vi "Localization - Read and Parse File.vi"(8 "Error In":errorcluster, 9 "Full File Contents in":string[][](array[string]), 10 "Localization File Path":path=path "C:/Apps/Dev/CMC Internal/Team Tools/Development/Composite Controls/Test VI/INI Files/Test.ini" caption="Localization File for Referenced VI", 11 "VI Reference":refnum<vi>) -> (0 "Error Out":errorcluster, 1 "Full File Contents out":string[][](array[string]), 2 "Controls Not Present":string[](array[string]), 3 "Array":refnum<class "Control Info.lvclass">[](array[class]))   [LabVIEW 2017, in "Localization.lvlib"]
uses:
  Localization.lvlib
  Control Info/Control Info.lvclass
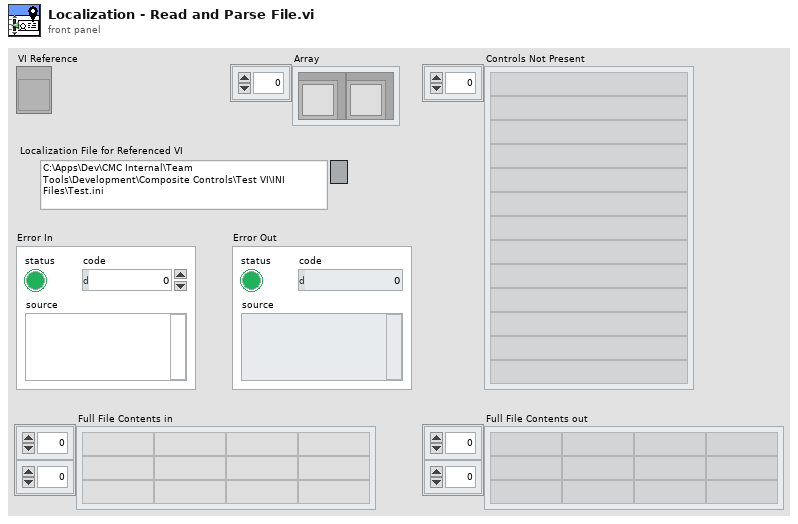
[diagram p1: front panel]
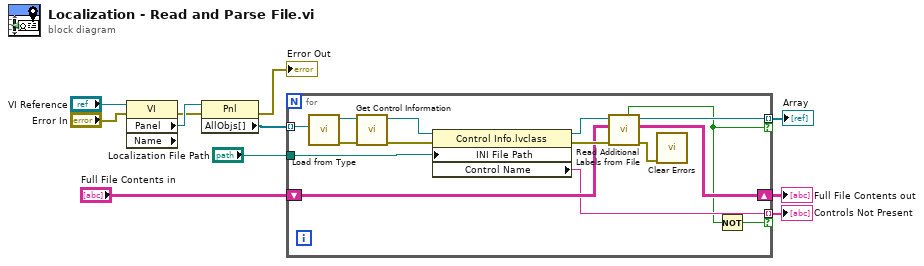
[diagram p0: block diagram]
diagram:
  n1 = property class="VI" props=["Panel", "Name"](reference="VI Reference", error in="Error In") -> (error out=w7:errorcluster, "Panel"=w8:refnum<vi>)  [unwired: 2 out]
  n2 = property class="Pnl"(reference=w8, error in=w7) -> (error out=→"Error Out":errorcluster, "AllObjs[]"=w6:refnum<vi>[])  [unwired: 1 out]
  n3 = for {
    tunnel: w6 -> [w26] mode=indexing
    tunnel: "Localization File Path" -> [w19]
    tunnel: [w18] -> w10 mode=indexing if=w13
    shift-right: [w17] -> w1
    shift-left: "Full File Contents in" -> [w16]
    tunnel: [w14] -> w2 mode=indexing if=w12
    n4 = call "Load from Type.vi"("Control Reference"=w26) -> ("error out"=w25:errorcluster, "Control Info out"=w24:refnum<class "Control Info.lvclass">)  [unwired: 9 in]
    n5 = call-dynamic "Get Control Information.vi"("error in (no error)"=w25, "Control Info in"=w24) -> ("error out"=w22:errorcluster, "Control Info out"=w23:refnum<class "Control Info.lvclass">)  [unwired: 7 in, 1 out]
    n6 = property class="Control Info.lvclass"(reference=w23, error in=w22, "INI File Path"=w19) -> (reference out=w20:refnum<class "Control Info.lvclass">, error out=w21:errorcluster, "Control Name"=w14:string)
    n7 = call-dynamic "Read Additional Labels from File.vi"("error in (no error)"=w21, "Full File Contents in"=w16, "Control Info in"=w20) -> ("error out"=w15:errorcluster, "Full File Contents out"=w17:string[][], "Control Info out"=w18:refnum<class "Control Info.lvclass">, "Control Present in File"=w13:bool)  [unwired: 5 in]
    n8 = call <vilib>:"Clear Errors.vi"("error in (no error)"=w15) -> ()  [unwired: 5 in, 2 out]
    n9 = Not(x=w13) -> (.not. x?=w12:bool)
  }
  "Array" <- w10
  "Controls Not Present" <- w2
  "Full File Contents out" <- w1
